vi "DDS Pulse IO Reset.vi"(8 "error in (no error)":errorcluster, 11 "spi script reference in":T1) -> (0 "error out":errorcluster, 3 "spi script reference out":T1)   [LabVIEW 2013, in "DDS.lvlib"]
doc: "Pulses IO Reset on all boards as part of a USB-8451 script."
uses:
  DDS.lvlib
  <vilib>/ni845x/ni845x.llb/ni845xSpiScriptControl.ctl
  Controls/DDS CS pins.ctl
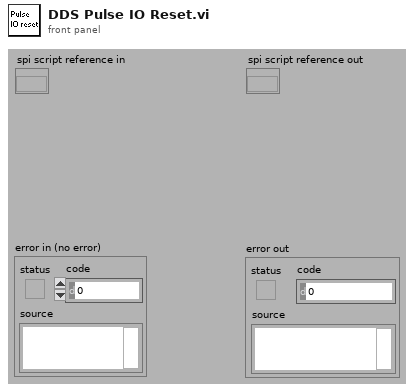
[diagram p1: front panel]
types:
  T1 = typedef "ni845xSpiScriptControl.ctl" = refnum<k20>
  T2 = typedef "DDS.lvlib/DDS CS pins.ctl" = enum8{"IO reset", "Ch. 4 CS", "Ch. 3 CS", "Ch. 2 CS", "Ch. 1 CS"}
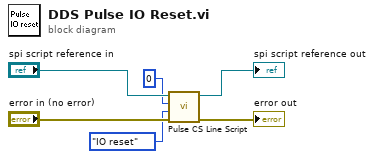
[diagram p0: block diagram]
diagram:
  n1 = call "Pulse CS Line Script.vi"("error in (no error)"="error in (no error)", "CS line number (0)"=DDS_CS_pins."IO reset" ("DDS CS pins"), "pulse width delay [ms] (0)"=u8 0, "spi script reference in"="spi script reference in") -> ("error out"=→"error out":errorcluster, "spi script reference out"=→"spi script reference out":T1)  [unwired: 6 in]
